vi "0-Draw Waypoints.vi"(4 "Image Descriptor":T6={"Upper-Left Corner Coordinates"={"UTM Zone"=0.0, "Hemisphere"=enum."North", "East"=0.0, "North"=0.0}, "Meters/Pixel"=42.294203}, 5 "Waypoints List":T2, 6 "Current Waypoint #":T1=-1, 7 "Image In":T7) -> (1 "Coordinate Outside Image":bool, 3 "Image Out":T7)   [LabVIEW 2011]
doc: "Overlays waypoints onto the map image."
uses:
  <vilib>/vision/Image Controls.llb/IMAQ Image.ctl
  0-Image Descriptor.ctl
  2-Think/2 Typedefs/UTM Location.ctl
  0x2-OCU-Think Comm/0x2 Typedefs/Waypoints List.ctl
  0x2-OCU-Think Comm/0x2 Typedefs/ocuWaypoint.ctl
  0x2-OCU-Think Comm/0x2 Typedefs/waypointTypes.ctl
  0x2-OCU-Think Comm/0x2 Typedefs/Current Waypoint.ctl
panel:
  in  "Current Waypt Color":u32(colorbox)=1985280
  in  "Finished Waypt Color":u32(colorbox)=57855
  in  "Waypt Color":u32(colorbox)=16711680
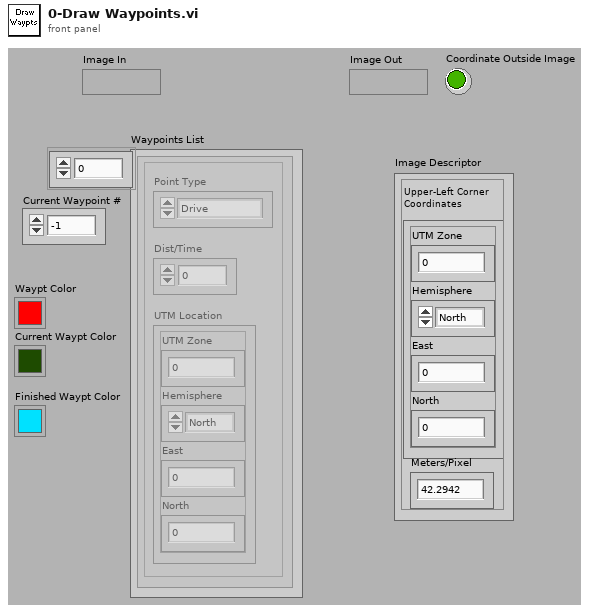
[diagram p1: front panel]
types:
  T1 = typedef "Current Waypoint.ctl" = i32
  T2 = typedef "Waypoints List.ctl" = T3[]
  T3 = typedef "ocuWaypoint.ctl" = cluster{"Point Type":T4, "Dist/Time":dbl, "UTM Location":T5}
  T4 = typedef "waypointTypes.ctl" = enum16{"Drive", "Round Port", "Round Starboard", "Stay"}
  T5 = typedef "UTM Location.ctl" = cluster{"UTM Zone":dbl, "Hemisphere":enum16{"North", "South"}, "East":dbl, "North":dbl}
  T6 = typedef "0-Image Descriptor.ctl" = cluster{"Upper-Left Corner Coordinates":T5, "Meters/Pixel":dbl}
  T7 = typedef "IMAQ Image.ctl" = refnum<image>
  T8 = cluster{"Desired Font (Application)":enum16{"User-specified Font", "Application Font", "System Font", "Dialog Font"}, "[User-specified Font]":cluster{"Font Name":string, "Size":i16, "Strikeout?":bool, "Italic?":bool, "Underline?":bool, "Outline?":bool, "Shadow?":bool, "Bold?":bool, "Rotation Angle":dbl}, "Horizontal Alignment":i16, "Vertical Alignment":i16}
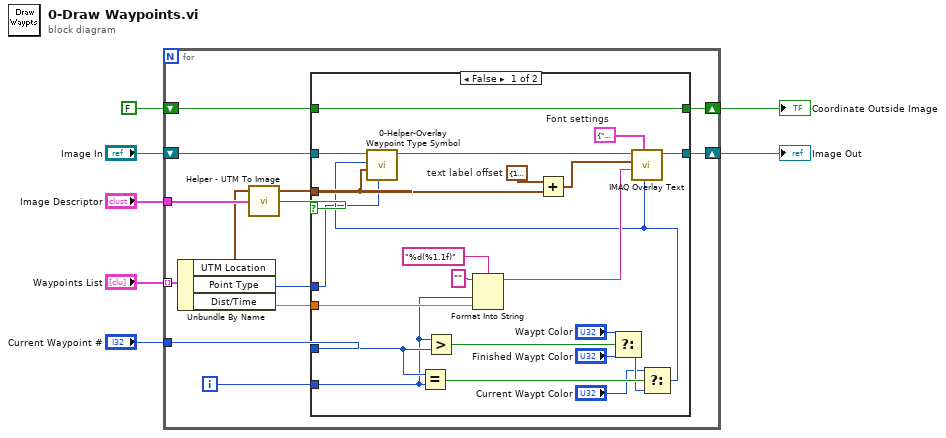
[diagram p0: block diagram]
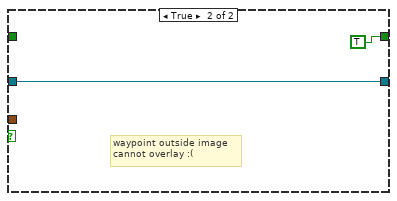
[diagram p2: hidden frame]
diagram:
  n1 = for {
    tunnel: "Waypoints List" -> [w17] mode=indexing
    shift-right: [w19] -> w6
    shift-left: "Image In" -> [w20]
    tunnel: "Image Descriptor" -> [w18]
    tunnel: "Current Waypoint #" -> [w13]
    shift-right: [w10] -> w2
    shift-left: FALSE -> [w9]
    i -> [w8]
    n2 = Unbundle By Name(w17) -> ("UTM Location"=w16:T5, "Point Type"=w14:T4, "Dist/Time"=w15:dbl)
    n3 = call "Helper - UTM To Image.vi"("Image Descriptor"=w18, "UTM Location"=w16) -> ("Coordinate Outside Image"=w11:bool, "Pixel Coordinates"=w12:cluster{"X":i32, "Y":i32})  [unwired: 1 in, 1 out]
    n4 = case shown="False" w11 {
      tunnel: w20 -> [w27 w44]
      tunnel: [w39 w44] -> w19
      tunnel: w15 -> [w22 _]
      tunnel: w14 -> [w24 _]
      tunnel: w13 -> [w34 _]
      tunnel: w12 -> [w26 _]
      tunnel: [w29 TRUE] -> w10
      tunnel: w9 -> [w29 _]
      tunnel: w8 -> [w21 _]
      frame False {
        w42 = T8 {"Desired Font (Application)"=enum."User-specified Font", "[User-specified Font]"={"Font Name"="Arial Unicode MS", "Size"=40, "Strikeout?"=FALSE, "Italic?"=FALSE, "Underline?"=FALSE, "Outline?"=FALSE, "Shadow?"=FALSE, "Bold?"=TRUE, "Rotation Angle"=0.0}, "Horizontal Alignment"=0, "Vertical Alignment"=0}  # Font settings
        w41 = cluster{"X":i32, "Y":i32} {"X"=10, "Y"=21}  # text label offset
        n5 = Equal?(x=w34, y=w21) -> (x = y?=w33:bool)
        n6 = Greater?(x=w21, y=w34) -> (0:w37:bool)
        n7 = Format Into String(format string="%d(%1.1f)", initial string="", w21, w22) -> (resulting string=w30:string)  [unwired: 1 in, 1 out]
        n8 = Add(x=w41, y=w26) -> (x+y=w40:cluster{"X":i32, "Y":i32})
        n9 = Select(t="Waypt Color", s=w37, f="Finished Waypt Color") -> (s? t:f=w32:u32)
        n10 = Select(t="Current Waypt Color", s=w33, f=w32) -> (s? t:f=w25:u32)
        n11 = call "0-Helper-Overlay Waypoint Type Symbol.vi"("Point Type"=w24, "Overlay Location"=w26, "Icon Color"=w25, "Image in"=w27) -> ("Image out"=w28:T7)  [unwired: 6 in, 1 out]
        n12 = call "IMAQ Overlay Text"("Text Color (black)"=w25, "Font, Size & Style"=w42, "String"=w30, "Origin"=w40, "Image"=w28) -> ("Image Out"=w39:T7)  [unwired: 3 in, 3 out]
      }
      frame True {
        # "waypoint outside image\ncannot overlay :("
      }
    }
  }
  "Image Out" <- w6
  "Coordinate Outside Image" <- w2
